vi "Query Channel Characteristics.vi"(8 "error in (no error)":errorcluster, 11 "VISA resource name":refnum<visa-resource-name>) -> (0 "error out":errorcluster, 1 "Trigger Level":dbl, 2 "Impedance":dbl, 3 "VISA resource name out":refnum<visa-resource-name>, 4 "Slope":u32(ring) items=["Positive", "Negative"], 5 "Coupling":u32(ring) items=["AC", "DC"], 7 "Cutoff Frequency":dbl)   [LabVIEW 2020, in "Counter.lvlib" / "PICOTEST U62XXA series.lvlib"]
doc: "Returns Channel 3 characteristics <B>(for U6200A model only)</B>.\n\n<B>Note:</B>\n\nThis VI should only be called if Option 030/050 is installed.\nOption 030, 3.0 GHz RF Input Channel (Channel 3)\nOption 050, 5.0 GHz RF Input Channel (Channel 3)"
uses:
  PICOTEST U62XXA series.lvlib
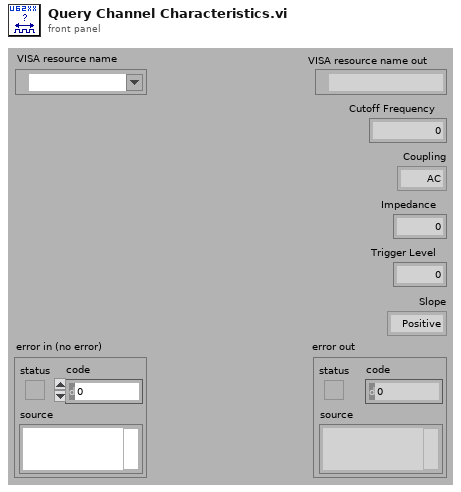
[diagram p1: front panel]
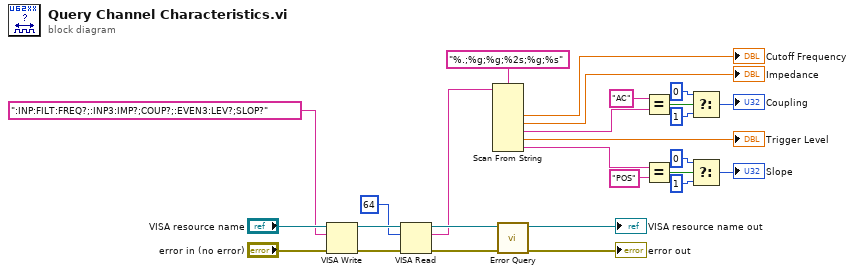
[diagram p0: block diagram]
diagram:
  n1 = VISA Write(VISA resource name="VISA resource name", write buffer=":INP:FILT:FREQ?;:INP3:IMP?;COUP?;:EVEN3:LEV?;SLOP?", error in (no error)="error in (no error)") -> (VISA resource name out=w27:refnum<visa-resource-name>, error out=w26:errorcluster)  [unwired: 1 out]
  n2 = VISA Read(VISA resource name=w27, byte count=u32 64, error in (no error)=w26) -> (VISA resource name out=w22:refnum<visa-resource-name>, read buffer=w8:string, error out=w21:errorcluster)  [unwired: 1 out]
  n3 = Scan From String(format string="%.;%g;%g;%2s;%g;%s", input string=w8) -> (output 1=→"Cutoff Frequency":dbl, output 2=→"Impedance":dbl, output 3=w6:string, output 4=→"Trigger Level":dbl, output 5=w4:string)  [unwired: 7 in, 3 out]
  n4 = call "Error Query.vi"("error in (no error)"=w21, "VISA resource name"=w22) -> ("error out"=→"error out":errorcluster, "VISA resource name out"=→"VISA resource name out":refnum<visa-resource-name>)  [unwired: 6 in, 2 out]
  n5 = Equal?(x="AC" ("y"), y=w6) -> (x = y?=w18:bool)
  n6 = Equal?(x=w4, y="POS") -> (x = y?=w12:bool)
  n7 = Select(t=u32 0, s=w18, f=u32 1) -> (s? t:f=→"Coupling":u32)
  n8 = Select(t=u32 0, s=w12, f=u32 1) -> (s? t:f=→"Slope":u32)
